vi "Save As TIFF.vi"(6 "Camera Type":T1, 8 "error in (no error)":errorcluster, 10 "Raw file paths":path[](array[path]), 11 "Camera in":refnum<class "Camera.lvclass">) -> (0 "error out":errorcluster, 3 "Camera out":refnum<class "Camera.lvclass">)   [LabVIEW 2023, in "Camera.lvlib" / "Camera.lvclass"]
uses:
  Camera.lvclass
  Resources/Type Defs/Camera Type.ctl
  Camera.lvclass/Camera.ctl
  Tiff Writer/Tiff Writer Messages/Save Tiff Msg/Save Tiff Msg.lvclass/Save Tiff Msg.ctl
  <vilib>/ActorFramework/Message Enqueuer/Message Enqueuer.lvclass/Message Enqueuer.ctl
  <vilib>/ActorFramework/Message Enqueuer/Enqueue.vi
  Tiff Writer/Tiff Writer Messages/Save Tiff Msg/Save Tiff Msg.lvclass
  Resources/GLOBAL/GLOBAL Experiment Metadata.vi
  Resources/GLOBAL/GLOBAL Time-critical.vi
  <vilib>/ActorFramework/Message Priority Queue/Priority Enqueue.vi
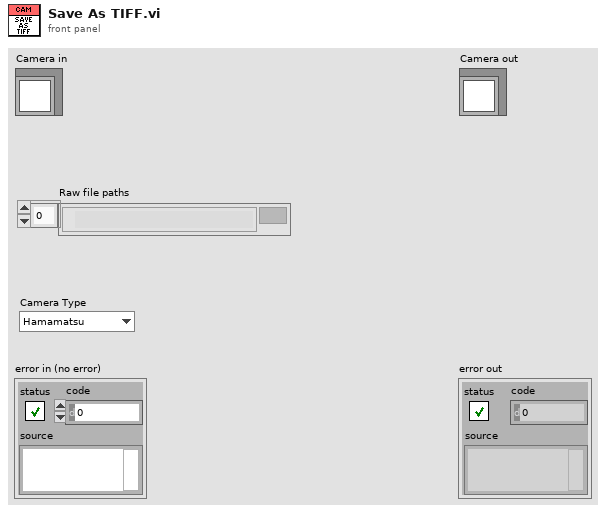
[diagram p1: front panel]
types:
  T1 = typedef "Camera Type.ctl" = enum16{"Hamamatsu", "Andor", "Photometrics"}
  T2 = typedef "Camera Settings.ctl" = cluster{"Exposure Time (ms)":dbl, "Binning":enum16{"1x1", "2x2", "4x4"}, "Scan Mode":i32, "Frames to Acquire":dbl, "Pixel Correction":bool, "Frames to Skip":u32, "File Path":path, "Duty cycle":dbl, "ALEX":bool, "Shutter Enable":bool[], "fluidics trigger frame":u16, "Bit Depth":u16, "Image Width (px)":u16, "Image Height (px)":u16, "Horizontal Offset (px)":u16, "Vertical Offset (px)":u16}
  T3 = typedef "Stack Info.ctl" = cluster{"Number of Frames":u32, "Image Width (px)":u32, "Image Height (px)":u32, "Pixel Size (nm)":dbl, "Exposure Time (ms)":dbl, "Frame Time (ms)":dbl, "Number of Channels":u32, "Bit Depth":u32, "Image Description":string, "Camera Type":T1}
  T4 = typedef "Physical Camera Assignment.ctl" = cluster{"Channel Name":string, "Serial Number":string, "Flip Vertically":bool, "Flip Horizontally":bool, "wavelength":i16, "photonsPerCount":dbl[]}
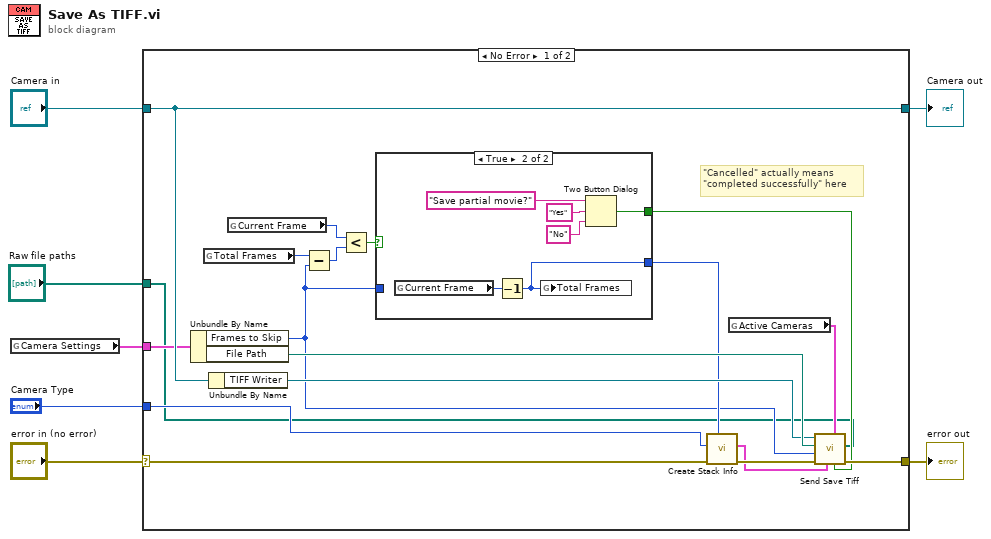
[diagram p0: block diagram]
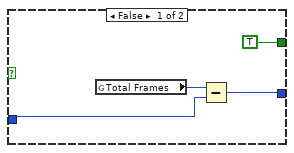
[diagram p2: hidden frame]
diagram:
  n1 = global read "GLOBAL Experiment Metadata.vi" "Camera Settings"() -> (w3:T2)
  n2 = case shown="No Error" "error in (no error)" {
    selector: "error in (no error)" -> [w24 w37]
    tunnel: [w25 w37] -> w6
    tunnel: [w22 w36] -> w4
    tunnel: "Camera in" -> [w22 w36]
    tunnel: w3 -> [w12 _]
    tunnel: "Camera Type" -> [w20 _]
    tunnel: "Raw file paths" -> [w8 _]
    frame No Error {
      # "\"Cancelled\" actually means\n\"completed successfully\" here"
      n3 = Unbundle By Name(w12) -> ("Frames to Skip"=w13:u32, "File Path"=w23:path)
      n4 = global read "GLOBAL Time-critical.vi" "Total Frames"() -> (w18:i32)
      n5 = Unbundle By Name(w22) -> ("TIFF Writer"=w21:refnum<class "Message Enqueuer.lvclass">)
      n6 = global read "GLOBAL Time-critical.vi" "Current Frame"() -> (w17:i32)
      n7 = Subtract(x=w18, y=w13) -> (x-y=w19:u32)
      n8 = Less?(x=w17, y=w19) -> (x < y?=w16:bool)
      n9 = case shown="True" w16 {
        tunnel: [TRUE ("T button?") w32] -> w15
        tunnel: [w26 w31] -> w14
        tunnel: w13 -> [w27 _]
        frame False {
          n10 = global read "GLOBAL Time-critical.vi" "Total Frames"() -> (w28:i32)
          n11 = Subtract(x=w28, y=w27) -> (x-y=w26:u32)
        }
        frame True {
          n12 = global read "GLOBAL Time-critical.vi" "Current Frame"() -> (w30:i32)
          n13 = Decrement(x=w30) -> (x-1=w31:i32)
          n14 = global write "GLOBAL Time-critical.vi" "Total Frames"(w31) -> ()
          n15 = Two Button Dialog(message="Save partial movie?", 1:"No" ("F button name (\"Cancel\")"), 2:"Yes" ("T button name (\"OK\")")) -> (T button?=w32:bool)
        }
      }
      n16 = call "Create Stack Info.vi"("nFrames"=w14, "error in (no error)"=w24, "Camera Type"=w20) -> ("error out"=w10:errorcluster, "Stack Info"=w9:T3)  [unwired: 7 in]
      n17 = global read "GLOBAL Time-critical.vi" "Active Cameras"() -> (w11:T4[])
      n18 = call "Send Save Tiff.vi"("Raw file paths"=w8, "Cancelled"=w15, "Active Cameras"=w11, "Stack Info"=w9, "error in (no error)"=w10, "Frames to Skip"=w13, "File Path"=w23, "Message Enqueuer"=w21) -> ("error out"=w25:errorcluster)  [unwired: 2 in, 1 out]
    }
    frame Error {
    }
  }
  "error out" <- w6
  "Camera out" <- w4
